vi "Dashboard Main.vi"() -> ()   [LabVIEW 2013]
uses:
  <vilib>/event_ctls.llb/eventvkey.ctl
  <vilib>/Rock Robotics/WPI/Dashboard/WPI_DashboardLogging Global.vi
  <vilib>/Utility/config.llb/Write Key (String).vi
  <vilib>/Utility/config.llb/Write Key (I32).vi
  <vilib>/Utility/config.llb/NI_LVConfig.lvlib
panel:
  out "Image Message":string="Timeout in Camera Communications"
  in  "Rec Mode":enum32{"Stop", "Record", "Playback"}(radio)
  in  "Dashboard Tab":T1(tab)
  out "Limit Switches":T2
  in  "Camera Settings":T3={"Frame Rate"=30, "Compression"=30, "Size"=1} {"Frame Rate" scale=1.0..30.0; "Size" items=["640x480", "320x240", "160x120"]}
  out "MotorSliders R":cluster{"MotorSlide1":dbl, "MotorSlide2":dbl} {"MotorSlide2" scale=-1.0..1.0 scale format="%#_2e"; "MotorSlide1" scale=-1.0..1.0 scale format="%#_2e"}
  out "MotorChart R":cluster{"Numeric":dbl, "Numeric":dbl}(graph)
  out "MotorSliders L":T4 {"MotorSlide4 2" scale=0.0..14.0 scale format="%#_2e"; "MotorSlide2" scale=-1.0..1.0 scale format="%#_2e"; "MotorSlide1" scale=-1.0..1.0 scale format="%#_2e"}
  out "MotorChart L":T5(graph)
  out "JS1 Z":dbl(slide) scale=-1.0..1.0 scale format="%#_2e"
  out "Joystick 1":cluster{"X":dbl, "Y":dbl}[](graph)
  out "JS Buttons 1":T6
  out "JS2 Z":dbl(slide) scale=-1.0..1.0 scale format="%#_2e"
  out "Joystick 2":cluster{"X":dbl, "Y":dbl}[](graph)
  out "JS Buttons 2":T6
  out "Mode":T7(ring)=enum."Auto Disabled"
  out "Camera IP":string
  in  "DB Camera Config":bool
  out "fps":dbl format="%#.1g"
  out "Mbps":dbl format="%#.1g"
  out "Mbps 2":bool
  out "LED 1":bool
  out "Gamepad JS 1":cluster{"X":dbl, "Y":dbl}[](graph)
  out "Gamepad Buttons":T6
  out "Gamepad Triggers":dbl(slide) scale=-1.0..1.0 scale format="%#_2e"
  out "Gamepad JS 2":cluster{"X":dbl, "Y":dbl}[](graph)
  in  "C/J":bool
  in  "T/A":bool
  in  "Slider 1":dbl(slide) scale=0.0..100.0
  in  "Checkbox 2":bool
  in  "Checkbox 1":bool
  in  "Test Slider":dbl(slide) scale=0.0..100.0 scale format="%#_3g"
  in  "On/Off":bool caption="Solenoid"
  in  "Test Name":u16(ring) items=["Select the test to run...", "Example Test", "-------------------------------", "List of tests is built in robot code.", "Replace with your own automated tests."]
  in  "Test Tree":string(tree)
  in  "Motor":cluster{"Value":dbl, "Enable":bool} {"Value" scale=-1.0..1.0 scale format="%#_3g"}
  out "Progress":T8 {"Test Progress" scale=0.0..100.0}
  in  "Rev/Fwd":cluster{"Forward":bool, "Reverse":bool}
  in  "Test Ring":u16(ring) items=["Auto", "Fixed indoor", "Fixed outdoor 1", "Fixed outdoor 2", "Fixed fluorescent 1", "Fixed fluorescent 2", "Hold current"]
  in  "Listbox":i32(listbox)
  out "Tree":string(tree)
  out "Camera Image":T9(plugin-control)
  in  "Enable":bool
  # "Gamepad 1"
  # "Joystick 1"
  # "Joystick 2"
  # "Left"
  # "Front"
  # "Right"
  # "Battery"
  # "Customize by placing controls and indicators here and name to\nmatch Dashboard Variables on robot."
  # "This tab is a great place for autonomous settings and validation.\nCustomize by placing controls and indicators here and name to\nmatch Dashboard Variables on robot."
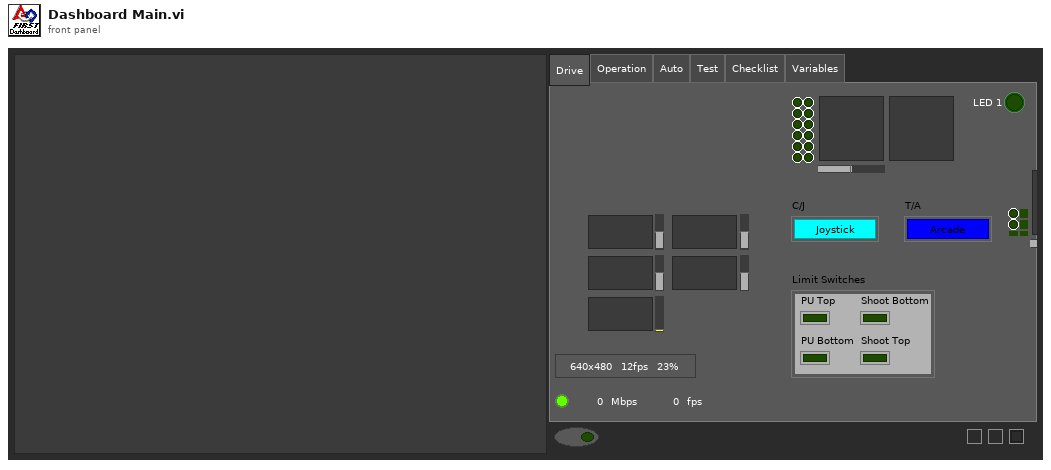
[diagram p1: front panel]
types:
  T1 = enum32{"Drive", "Operation", "Auto", "Test", "Checklist", "Variables"}
  T2 = cluster{"PU Top":bool, "PU Bottom":bool, "Shoot Bottom":bool, "Shoot Top":bool}
  T3 = cluster{"Frame Rate":i32, "Compression":i32, "Size":u16}
  T4 = cluster{"MotorSlide1":dbl, "MotorSlide2":dbl, "MotorSlide4 2":dbl}
  T5 = cluster{"Numeric":dbl, "Numeric":dbl, "Battery":sgl}
  T6 = cluster{bool, bool, bool, bool, bool, bool, bool, bool, bool, bool, bool, bool}
  T7 = enum8{"Tele-Op Disabled", "Tele-Op Enabled", "Auto Disabled", "Auto Enabled", "Test Disabled", "Test Enabled", ""}
  T8 = cluster{"Test Progress":u8, "Test Progress Text":string}
  T9 = typedef "IMAQ Image.ctl" = refnum<image>
  T10 = typedef "Image Type" = u32
  T11 = cluster{"Digital Inputs":bool[], "Digital Outputs":bool[]}
  T12 = cluster{"Competition mode":bool, "Robot Link":bool, "Autonomous":bool, "Enabled":bool, "E-Stop":bool, "Simulated":bool, "TestMode":bool, "Docked Window":bool}
  T13 = cluster{"Boolean Array[0]":bool, "Boolean Array[1]":bool, "Boolean Array[2]":bool, "Boolean Array[3]":bool, "Boolean Array[4]":bool, "Boolean Array[5]":bool, "Boolean Array[6]":bool, "Boolean Array[7]":bool, "Boolean Array[8]":bool, "Boolean Array[9]":bool, "Boolean Array[10]":bool, "Boolean Array[11]":bool}
  T14 = cluster{"Boolean Array[0]":bool, "Boolean Array[1]":bool, "Boolean Array[2]":bool, "Boolean Array[3]":bool}
  T15 = typedef "NI_LVConfig.lvlib/Config Data RefNum.ctl" = refnum<k1>
  T16 = typedef "eventvkey.ctl" = enum16{"ASCII", "Enter", "Return", "Shift", "Ctrl", "Alt", "Cmd", "Opt", "Caps", "NumLock", "Clear", "Break", "Up", "Down", "Left", "Right", "Insert", "Delete", "Home", "End", "PageUp", "PageDown", "Escape", "Help", "Pause", "ScrollLock", "F1", "F2", "F3", "F4", "F5", "F6", "F7", "F8", "F9", "F10", "F11", "F12", "F13", "F14", "F15", "F16", "F17", "F18", "F19", "F20", "F21", "F22", "F23", "F24", "Play", "VolumeUp", "VolumeDown", "Mute", "Two Byte Char"}
  T17 = cluster{"Image Size":bool, "Image Type":bool, "Pixel Value":bool, "ROI Information":bool, "Zoom Factor":bool}
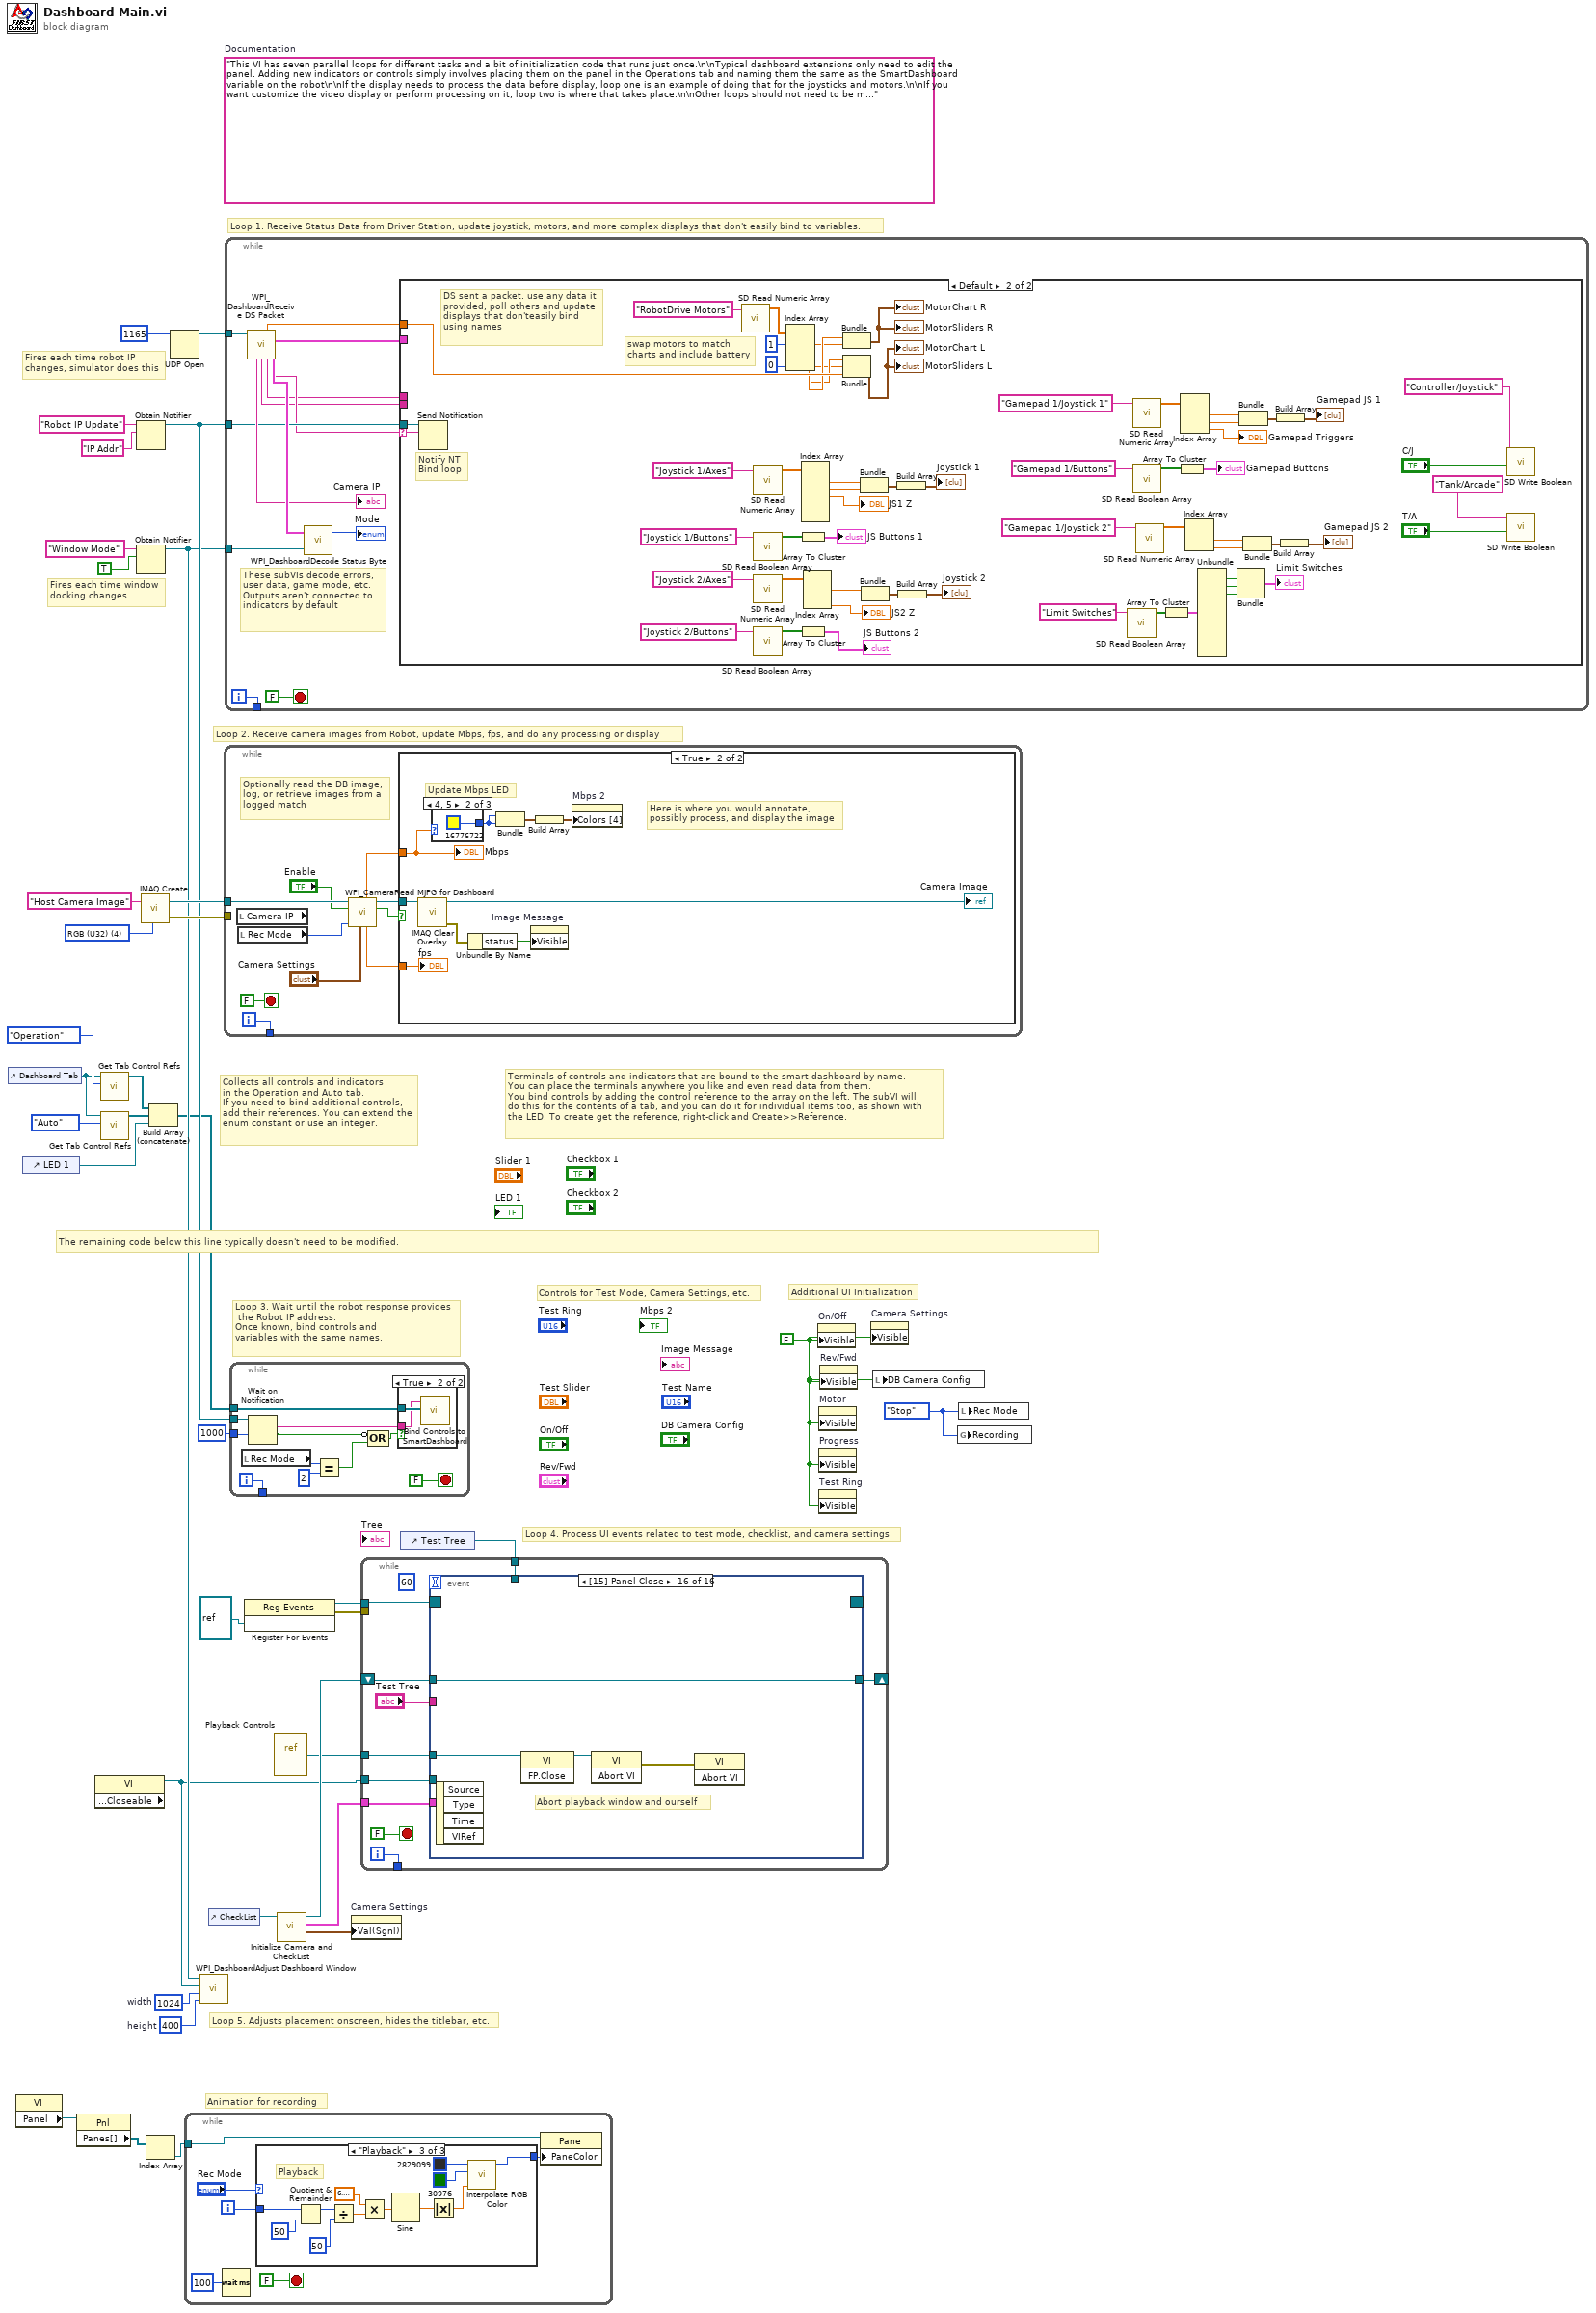
[diagram p0: block diagram]
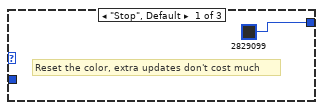
[diagram p2: hidden frame]
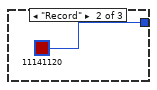
[diagram p3: hidden frame]
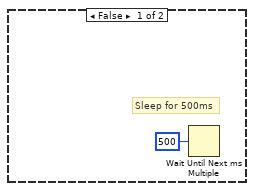
[diagram p5: hidden frame]
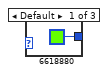
[diagram p6: hidden frame]
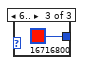
[diagram p7: hidden frame]
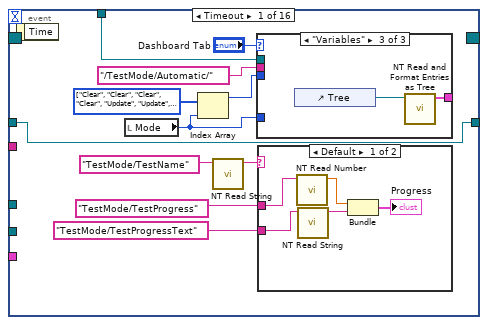
[diagram p8: hidden frame]
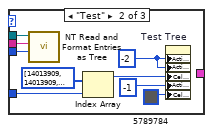
[diagram p10: hidden frame]
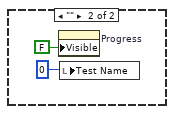
[diagram p11: hidden frame]
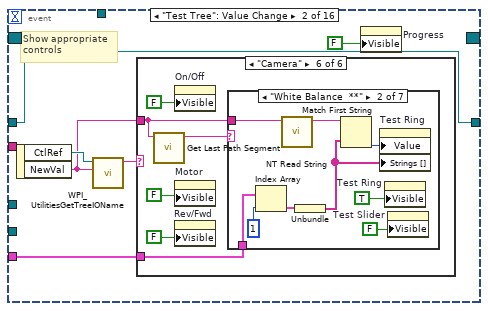
[diagram p12: hidden frame]
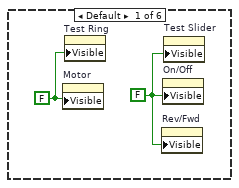
[diagram p13: hidden frame]
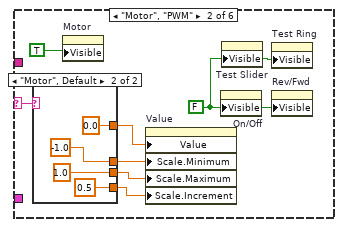
[diagram p14: hidden frame]
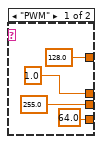
[diagram p15: hidden frame]
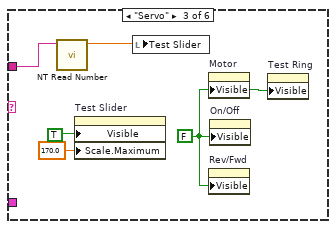
[diagram p16: hidden frame]
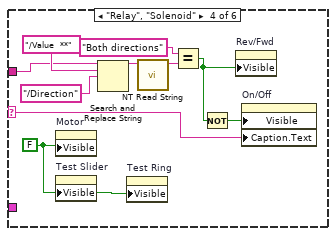
[diagram p17: hidden frame]
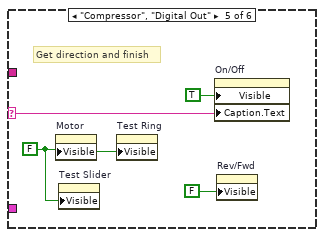
[diagram p18: hidden frame]
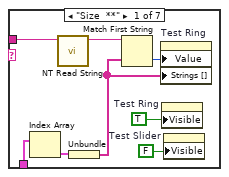
[diagram p19: hidden frame]
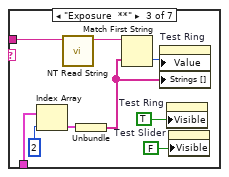
[diagram p20: hidden frame]
diagram:
  w8 = enum32{"Stop", "Record", "Playback"}."Stop" ("Rec Mode")
  w11 = 400  # height
  w12 = 1024  # width
  w25 = FALSE ("Visible")
  (unwired) "This VI has seven parallel loops for different tasks and a bit of initialization code that runs just once.\n\nTypical dashboard extensions only need to edit the panel. Adding new indicators or controls simply involves placing them on the panel in the Operations tab and naming them the same as the SmartDashboard variable on the robot\n\nIf the display needs to process the data before display, loop one is an example of doing that for the joysticks and motors.\n\nIf you want customize the video display or perform processing on it, loop two is where that takes place.\n\nOther loops should not need to be modified. They are pretty standard, and document the task they perform."  # Documentation
  w35 = T10 4 items=["Grayscale (U8)", "Grayscale (I16)", "Grayscale (SGL)", "Complex (CSG)", "RGB (U32)", "HSL (U32)", "RGB (U64)"] ("Image Type")
  # "Controls for Test Mode, Camera Settings, etc."
  # "Additional UI Initialization"
  # "Animation for recording"
  # "Fires each time robot IP\nchanges, simulator does this"
  # "Fires each time window\ndocking changes."
  # "Collects all controls and indicators\nin the Operation and Auto tab.\nIf you need to bind additional controls,\nadd their references. You can extend the\nenum constant or use an integer."
  # "The remaining code below this line typically doesn't need to be modified."
  # "Loop 4. Process UI events related to test mode, checklist, and camera settings"
  # "Terminals of controls and indicators that are bound to the smart dashboard by name.\nYou can place the terminals anywhere you like and even read data from them.\nYou bind controls by adding the control reference to the array on the left. The subVI will\ndo this for the contents of a tab, and you can do it for individual items too, as shown with\nthe LED. To create get the reference, right-click and Create>>Reference."
  # "Loop 3. Wait until the robot response provides\n the Robot IP address.\nOnce known, bind controls and\nvariables with the same names."
  # "Loop 5. Adjusts placement onscreen, hides the titlebar, etc."
  # "Loop 1. Receive Status Data from Driver Station, update joystick, motors, and more complex displays that don't easily bind to variables."
  # "Loop 2. Receive camera images from Robot, update Mbps, fps, and do any processing or display"
  n1 = control-ref of="Dashboard Tab"() -> (w6:refnum<vi>)
  n2 = property class="VI"() -> ("Panel"=w19:refnum<vi>)  [unwired: 2 in, 2 out]
  n3 = control-ref of="LED 1"() -> (w1:refnum<vi>)
  n4 = property class="Pnl"(reference=w19) -> ("Panes[]"=w20:refnum<vi>[])  [unwired: 1 in, 2 out]
  n5 = property class="VI" props=["Front Panel.Closeable"]() -> (reference out=w7:refnum<vi>)  [unwired: 2 in, 2 out]
  n6 = call <vilib>:"Get Tab Control Refs.vi"("Page Index"=T1."Operation" ("Dashboard Tab"), "TabControl in"=w6) -> ("ControlsOnPage"=w4:refnum<vi>[])  [unwired: 9 in]
  n7 = call <vilib>:"Get Tab Control Refs.vi"("Page Index"=T1."Auto" ("Dashboard Tab"), "TabControl in"=w6) -> ("ControlsOnPage"=w5:refnum<vi>[])  [unwired: 9 in]
  n8 = Obtain Notifier(name (unnamed)="Robot IP Update", notification data type="IP Addr" ("name (unnamed)")) -> (notifier out=w29:refnum<notifier>)  [unwired: 2 in, 2 out]
  n9 = Obtain Notifier(name (unnamed)="Window Mode", notification data type=TRUE) -> (notifier out=w10:refnum<notifier>)  [unwired: 2 in, 2 out]
  n10 = call "IMAQ Create"("Image Name"="Host Camera Image", "Image Type"=w35) -> ("New Image"=w33:T9, "error out"=w32:errorcluster)  [unwired: 2 in, 1 out]
  n11 = Index Array(array=w20) -> (element=w18:refnum<vi>)  [unwired: 1 in]
  n12 = Build Array (concatenate)(w4, w5, w1) -> (w3:refnum<vi>[])
  n13 = UDP Open(11:u16 1165 ("port")) -> (port=w36:refnum<k16>)  [unwired: 2 in, 4 out]
  n14 = while {
    tunnel: w18 -> [w39]
    i -> [w42]
    stop <- FALSE stop-if-true
    n15 = Wait (ms)(milliseconds to wait=u32 100) -> ()  [unwired: 1 out]
    n16 = case shown="\"Playback\"" "Rec Mode" {
      tunnel: w42 -> [_ _ w57]
      tunnel: [u32 2829099 ("Base Color") u32 11141120 ("Target Color") w46] -> w38
      frame "Stop", Default {
        # "Reset the color, extra updates don't cost much"
      }
      frame "Record" {
      }
      frame "Playback" {
        # "Playback"
        n17 = Quotient & Remainder(x=w57, y=u32 50 ("milliseconds to wait")) -> (x-y*floor(x/y)=w53:u32)  [unwired: 1 out]
        n18 = Divide(x=w53, y=u32 50 ("milliseconds to wait")) -> (x/y=w50:dbl)
        n19 = Multiply(x=6.283185307179586, y=w50) -> (x*y=w55:dbl)
        n20 = Sine(x=w55) -> (sin(x)=w54:dbl)
        n21 = Absolute Value(x=w54) -> (abs(x)=w47:dbl)
        n22 = call "Interpolate RGB Color.vi"("Proportion"=w47, "Target Color"=u32 30976, "Base Color"=u32 2829099) -> ("Result Color"=w46:u32)  [unwired: 8 in]
      }
    }
    n23 = property class="Pane"(reference=w39, "PaneColor"=w38) -> ()  [unwired: 1 in, 2 out]
  }
  n24 = call <vilib>:"WPI_DashboardAdjust Dashboard Window.vi"("height"=w11, "width"=w12, "reference in"=w7, "Notifier in"=w10) -> ()  [unwired: 8 in]
  n25 = control-ref of="CheckList"() -> (w9:refnum<vi>)
  n26 = while {
    tunnel: w33 -> [w66]
    tunnel: w32 -> [_]
    tunnel: [w67] -> _
    i -> [w67]
    stop <- FALSE stop-if-true
    # "Optionally read the DB image,\nlog, or retrieve images from a\nlogged match"
    n27 = local read "Camera IP"() -> (w59:string)
    n28 = local read "Rec Mode"() -> (w58:enum32{"Stop", "Record", "Playback"})
    n29 = call <vilib>:"WPI_CameraRead MJPG for Dashboard.vi"("Camera Settings"="Camera Settings", "Rec Mode"=w58, "Camera IP"=w59, "Enable"="Enable", "Refnum in"=w66) -> ("Active"=w63:bool, "Refnum out"=w65:T9, "FPS"=w62:dbl, "Bandwidth (Mbps)"=w61:dbl)  [unwired: 3 in]
    n30 = case shown="True" w63 {
      tunnel: w65 -> [_ w73]
      tunnel: w61 -> [_ w72]
      tunnel: w62 -> [_ w70]
      frame False {
        # "Sleep for 500ms"
        n31 = Wait Until Next ms Multiple(millisecond multiple=u32 500) -> ()  [unwired: 1 out]
      }
      frame True {
        # "Here is where you would annotate,\npossibly process, and display the image"
        # "Update Mbps LED"
        n32 = call "IMAQ Clear Overlay"("Image"=w73) -> ("error out"=w77:errorcluster, "Image Out"=→"Camera Image":T9)  [unwired: 2 in, 7 out]
        n33 = case shown="4, 5" w72 {
          tunnel: [u32 6618880 ("Color Box") u32 16776722 ("Color Box") u32 16716800 ("Color Box")] -> w74
          frame Default {
          }
          frame 4, 5 {
          }
          frame 6.. {
          }
        }
        n34 = Unbundle By Name(w77) -> ("status"=w78:bool)
        n35 = Bundle("Color Box"=w74, "Color Box"=w74) -> (w76:cluster{"Color Box":u32, "Color Box":u32})  [unwired: 1 out]
        n36 = property on="Image Message" class="Str"("Visible"=w78) -> ()  [unwired: 2 in, 2 out]
        n37 = Build Array(w76) -> (w75:cluster{"Color Box":u32, "Color Box":u32}[])
        n38 = property on="Mbps 2" class="Bool (strict)"("Colors [4]"=w75) -> ()  [unwired: 2 in, 2 out]
        "Mbps" <- w72
        "fps" <- w70
      }
    }
  }
  n39 = while {
    tunnel: w36 -> [w92]
    tunnel: w29 -> [w87]
    tunnel: w10 -> [w91]
    tunnel: [w88] -> _
    i -> [w88]
    stop <- FALSE stop-if-true
    # "These subVIs decode errors, user data, game mode, etc.\nOutputs aren't connected to indicators by default"
    n40 = call <vilib>:"WPI_DashboardReceive DS Packet.vi"("Recv Socket"=w92) -> ("Battery"=w82:sgl, "Driver Station"=w83:T11, "Robot IP Address"=w86:string, "Status"=w93:T12, "Camera IP Address"=→"Camera IP":string, "Low Priority User Data"=w85:string, "High Priority User Data"=w84:string)  [unwired: 1 in, 7 out]
    n41 = call <vilib>:"WPI_DashboardDecode Status Byte.vi"("Window Mode Notifier"=w91, "Status"=w93) -> ("Mode"=→"Mode":T7)  [unwired: 1 out]
    n42 = case shown="Default" w86 {
      selector: w86 -> [_ w133]
      tunnel: w87 -> [_ w134]
      tunnel: w85 -> [_ _]
      tunnel: w84 -> [_ _]
      tunnel: w83 -> [_ _]
      tunnel: w82 -> [_ w132]
      frame "0.0.0.0" {
        # "DS not sending packets, or no robot exists yet.\nDon't poll the variables"
      }
      frame Default {
        # "Notify NT\nBind loop"
        # "DS sent a packet. use any data it\nprovided, poll others and update\ndisplays that don'teasily bind\nusing names"
        # "swap motors to match\ncharts and include battery"
        n43 = Send Notification(notification=w133, notifier=w134) -> ()  [unwired: 1 in, 2 out]
        n44 = call <vilib>:"SD Read Numeric Array.vi"("Name"="RobotDrive Motors") -> ("Numeric Array"=w131:dbl[])  [unwired: 8 in, 2 out]
        n45 = call <vilib>:"SD Read Numeric Array.vi"("Name"="Joystick 1/Axes") -> ("Numeric Array"=w150:dbl[])  [unwired: 8 in, 2 out]
        n46 = call <vilib>:"SD Read Boolean Array.vi"("Name"="Joystick 1/Buttons") -> ("Boolean Array"=w152:bool[])  [unwired: 8 in, 2 out]
        n47 = call <vilib>:"SD Read Numeric Array.vi"("Name"="Joystick 2/Axes") -> ("Numeric Array"=w144:dbl[])  [unwired: 8 in, 2 out]
        n48 = call <vilib>:"SD Read Boolean Array.vi"("Name"="Joystick 2/Buttons") -> ("Boolean Array"=w143:bool[])  [unwired: 8 in, 2 out]
        n49 = Index Array(array=w131, index #1=1, index #4=0) -> (element #1=w127:dbl, element #2=w126:dbl, element #3=w128:dbl, element #4=w123:dbl)  [unwired: 2 in]
        n50 = Array To Cluster(array=w152) -> (cluster=→"JS Buttons 1":T13)
        n51 = Array To Cluster(array=w143) -> (cluster=→"JS Buttons 2":T13)
        n52 = Index Array(array=w150) -> (element #1=w147:dbl, element #2=w148:dbl, element #3=→"JS1 Z":dbl)  [unwired: 6 in, 3 out]
        n53 = Index Array(array=w144) -> (element #1=w139:dbl, element #2=w138:dbl, element #3=→"JS2 Z":dbl)  [unwired: 3 in]
        n54 = Bundle("Numeric"=w128, "Numeric"=w127) -> (→"MotorChart R" →"MotorSliders R":cluster{"Numeric":dbl, "Numeric":dbl})  [unwired: 1 in]
        n55 = Bundle("Numeric"=w126, "Numeric"=w123, "Battery"=w132) -> (→"MotorChart L" →"MotorSliders L":T5)  [unwired: 1 in]
        n56 = Bundle("Numeric"=w147, "Numeric"=w148) -> (w146:cluster{"Numeric":dbl, "Numeric":dbl})  [unwired: 1 in]
        n57 = Bundle("Numeric"=w139, "Numeric"=w138) -> (w140:cluster{"Numeric":dbl, "Numeric":dbl})  [unwired: 1 in]
        n58 = Build Array(w146) -> (→"Joystick 1":cluster{"Numeric":dbl, "Numeric":dbl}[])
        n59 = Build Array(w140) -> (→"Joystick 2":cluster{"Numeric":dbl, "Numeric":dbl}[])
        n60 = call <vilib>:"SD Read Boolean Array.vi"("Name"="Limit Switches") -> ("Boolean Array"=w105:bool[])  [unwired: 8 in, 2 out]
        n61 = call <vilib>:"SD Read Numeric Array.vi"("Name"="Gamepad 1/Joystick 1") -> ("Numeric Array"=w118:dbl[])  [unwired: 8 in, 2 out]
        n62 = call <vilib>:"SD Read Boolean Array.vi"("Name"="Gamepad 1/Buttons") -> ("Boolean Array"=w120:bool[])  [unwired: 8 in, 2 out]
        n63 = call <vilib>:"SD Read Numeric Array.vi"("Name"="Gamepad 1/Joystick 2") -> ("Numeric Array"=w112:dbl[])  [unwired: 8 in, 2 out]
        n64 = Array To Cluster(array=w105) -> (cluster=w104:T13)
        n65 = Array To Cluster(array=w120) -> (cluster=→"Gamepad Buttons":T13)
        n66 = Index Array(array=w118) -> (element #1=w115:dbl, element #2=w116:dbl, element #3=→"Gamepad Triggers":dbl)  [unwired: 3 in]
        n67 = Index Array(array=w112) -> (element #1=w109:dbl, element #2=w108:dbl)  [unwired: 2 in]
        n68 = Unbundle(w104) -> ("Boolean Array[0]"=w103:bool, "Boolean Array[1]"=w102:bool, "Boolean Array[2]"=w101:bool, "Boolean Array[3]"=w100:bool)  [unwired: 8 out]
        n69 = Bundle("Boolean Array[0]"=w103, "Boolean Array[1]"=w102, "Boolean Array[2]"=w101, "Boolean Array[3]"=w100) -> (→"Limit Switches":T14)  [unwired: 1 in]
        n70 = Bundle("Numeric"=w115, "Numeric"=w116) -> (w114:cluster{"Numeric":dbl, "Numeric":dbl})  [unwired: 1 in]
        n71 = Bundle("Numeric"=w109, "Numeric"=w108) -> (w110:cluster{"Numeric":dbl, "Numeric":dbl})  [unwired: 1 in]
        n72 = Build Array(w114) -> (→"Gamepad JS 1":cluster{"Numeric":dbl, "Numeric":dbl}[])
        n73 = Build Array(w110) -> (→"Gamepad JS 2":cluster{"Numeric":dbl, "Numeric":dbl}[])
        n74 = call <vilib>:"SD Write Boolean.vi"("Boolean"="C/J", "Name"="Controller/Joystick") -> ()  [unwired: 8 in, 2 out]
        n75 = call <vilib>:"SD Write Boolean.vi"("Boolean"="T/A", "Name"="Tank/Arcade") -> ()  [unwired: 8 in, 2 out]
      }
    }
  }
  n76 = while {
    tunnel: w3 -> [w166]
    tunnel: w29 -> [w164]
    tunnel: [w162] -> _
    tunnel: u32 1000 ("milliseconds to wait") -> [w161]
    i -> [w162]
    stop <- FALSE stop-if-true
    n77 = local read "Rec Mode"() -> (w157:enum32{"Stop", "Record", "Playback"})
    n78 = Wait on Notification(notifier=w164, timeout in ms (-1)=w161) -> (notification=w163:string, timed out?=w159:bool)  [unwired: 2 in, 2 out]
    n79 = Equal?(x=w157, y=u16 2 ("Rec Mode")) -> (x = y?=w158:bool)
    n80 = Compound Arithmetic op=OR(invert w159, w158) -> (w160:bool)
    n81 = case shown="True" w160 {
      tunnel: w166 -> [_ w168]
      tunnel: w163 -> [_ w167]
      frame False {
      }
      frame True {
        n82 = call <vilib>:"Bind Controls to SmartDashboard.vi"("Bound Control Refs"=w168, "Server IP Address"=w167) -> ()  [unwired: 10 in]
      }
    }
  }
  n83 = register-events(refnum<vi> refnum) -> (reference out=w16:refnum<event-registration>, error out=w15:errorcluster)  [unwired: 2 in]
  n84 = vi-ref "Playback Controls.vi"() -> (w17:refnum<vi>)
  n85 = call "Initialize Camera and CheckList.vi"("ListBox in"=w9) -> ("Cluster"=w23:cluster{"value":i32, "value":i32, "index":i32}, "Array"=w24:cluster{string[]}[], "File Refnum"=w22:T15)  [unwired: 8 in]
  n86 = property on="Camera Settings" class="Clust (strict)"("Val(Sgnl)"=w23) -> ()  [unwired: 2 in, 2 out]
  n87 = control-ref of="Test Tree"() -> (w21:refnum<vi>)
  n88 = while {
    tunnel: w24 -> [w176]
    shift-right: [w175] -> _
    shift-left: w22 -> [w174]
    tunnel: [w173] -> _
    tunnel: w21 -> [w172]
    tunnel: w17 -> [w171]
    tunnel: w16 -> [w170]
    tunnel: w15 -> [_]
    tunnel: w7 -> [w169]
    i -> [w173]
    stop <- FALSE stop-if-true
    n89 = event shown="[15] Panel Close" {
      selector: w170 -> [_ _ _ _ _ _ _ _ _ _ _ _ _ _ _ _]
      dyn-events: [_ _ _ _ _ _ _ _ _ _ _ _ _ w414 _ _] -> _
      timeout: u32 60 ("milliseconds to wait") -> [_ _ _ _ _ _ _ _ _ _ _ _ _ _ _ _]
      tunnel: w172 -> [w186 _ _ _ _ _ _ _ _ _ _ _ _ _ _ _]
      tunnel: "Test Tree" -> [_ _ _ _ _ _ _ _ w383 w391 w393 w397 w405 _ _ _]
      tunnel: w176 -> [_ w210 _ _ _ _ w347 w377 _ _ _ _ _ _ _ _]
      tunnel: [w180 w209 w308 w313 w321 w333 w346 w370 w382 w389 w392 w396 w404 w416 w430 w431] -> w175
      tunnel: w174 -> [w180 w209 w308 w313 w321 w333 w345 w370 w382 w389 w392 w396 w404 w416 w430 w431]
      tunnel: w171 -> [_ _ _ _ _ _ _ _ _ _ _ _ _ w417 _ w434]
      tunnel: w169 -> [_ _ _ _ _ _ _ _ _ _ _ _ _ w412 _ _]
      event Timeout {
        w185 = enum16{"Update", "Clear"}[] [enum."Clear", enum."Clear", enum."Clear", enum."Clear", enum."Update", enum."Update", enum."Clear"] items=["Update", "Clear"]
        n90 = event-data() -> ()  [unwired: 1 in, 1 out]
        n91 = local read "Mode"() -> (w183:T7)
        n92 = Index Array(array=w185, index=w183) -> (element=w184:enum16{"Update", "Clear"})
        n93 = call <vilib>:"NT Read String.vi"("Name"="TestMode/TestName") -> ("String"=w189:string)  [unwired: 9 in, 1 out]
        n94 = case shown="\"Variables\"" "Dashboard Tab" {
          tunnel: w186 -> [_ w199 _]
          tunnel: "/TestMode/Automatic/" ("Name Pattern") -> [_ w198 _]
          tunnel: w184 -> [_ w197 _]
          tunnel: w183 -> [_ w195 _]
          tunnel: [_ _ w201] -> _
          frame "Operation", Default {
          }
          frame "Test" {
            w194 = -2 ("Active Item:Row Number")
            n95 = call <vilib>:"NT Read and Format Entries as Tree.vi"("Operation"=w197, "Name Pattern"=w198, "Tree Refnum"=w199) -> ()  [unwired: 7 in, 2 out]
            n96 = Index Array(array=u32[] [14013909, 14013909, 14013909, 14013909, 14013909, 16777215, 14013909], index=w195) -> (element=w193:u32)
            n97 = property on="Test Tree" class="Tree (strict)"("Active Item Row Number"=w194, "ActiveColNum"=w194, "CellBG"=w193, "Active Item Row Number"=-1 ("Active Item:Row Number"), "CellBG"=u32 5789784 ("Color Box")) -> ()  [unwired: 2 in, 2 out]
          }
          frame "Variables" {
            n98 = control-ref of="Tree"() -> (w200:refnum<vi>)
            n99 = call <vilib>:"NT Read and Format Entries as Tree.vi"("Tree Refnum"=w200) -> ("Formatted Strings"=w201:cluster{"Name":string, "Value":string}[])  [unwired: 9 in, 1 out]
          }
        }
        n100 = case shown="Default" w189 {
          tunnel: "TestMode/TestProgress" ("Name") -> [w203 _]
          tunnel: "TestMode/TestProgressText" ("Name") -> [w202 _]
          frame Default {
            n101 = call <vilib>:"NT Read Number.vi"("Name"=w203) -> ("Numeric"=w204:dbl)  [unwired: 9 in, 1 out]
            n102 = call <vilib>:"NT Read String.vi"("Name"=w202) -> ("String"=w205:string)  [unwired: 9 in, 1 out]
            n103 = Bundle("Numeric"=w204, "String"=w205) -> (→"Progress":cluster{"Numeric":dbl, "String":string})  [unwired: 1 in]
          }
          frame "" {
            n104 = property on="Progress" class="Clust (strict)"("Visible"=FALSE) -> ()  [unwired: 2 in, 2 out]
            n105 = local write "Test Name"(u16 0) -> ()
          }
        }
      }
      event "Test Tree": Value Change {
        # "Show appropriate\ncontrols"
        n106 = event-data() -> ("CtlRef"=w213:refnum<vi>, "NewVal"=w211:string)  [unwired: 1 in]
        n107 = call <vilib>:"WPI_UtilitiesGetTreeIOName.vi"("NewVal"=w211, "TreeControl in"=w213) -> ("I/O Name"=w214:string)  [unwired: 9 in]
        n108 = case shown="\"Camera\"" w214 {
          selector: w214 -> [_ w221 _ w239 w248 _]
          tunnel: w211 -> [_ _ w236 w238 _ w255]
          tunnel: w210 -> [_ _ _ _ _ w254]
          frame Default {
            w216 = FALSE ("Visible")
            w215 = FALSE ("Visible")
            n109 = property on="Motor" class="Clust (strict)"("Visible"=w215) -> ()  [unwired: 2 in, 2 out]
            n110 = property on="Test Ring" class="Ring (strict)"("Visible"=w215) -> ()  [unwired: 2 in, 2 out]
            n111 = property on="Rev/Fwd" class="Clust (strict)"("Visible"=w216) -> ()  [unwired: 2 in, 2 out]
            n112 = property on="On/Off" class="Bool (strict)"("Visible"=w216) -> ()  [unwired: 2 in, 2 out]
            n113 = property on="Test Slider" class="Slide (strict)"("Visible"=w216) -> ()  [unwired: 2 in, 2 out]
          }
          frame "Motor", "PWM" {
            w222 = FALSE ("Visible")
            n114 = case shown="\"Motor\", Default" w221 {
              tunnel: [1.0 ("Value") -1.0 ("Value")] -> w220
              tunnel: [255.0 ("Value") 1.0 ("Value")] -> w219
              tunnel: [128.0 ("Value") 0.0 ("Value")] -> w218
              tunnel: [64.0 ("Value") 0.5 ("Value")] -> w217
              frame "PWM" {
              }
              frame "Motor", Default {
              }
            }
            n115 = property on="Motor" class="Clust (strict)"("Visible"=TRUE) -> ()  [unwired: 2 in, 2 out]
            n116 = property on="Value" class="Slide (strict)"("Value"=w218, "Scale.Minimum"=w220, "Scale.Maximum"=w219, "Scale.Increment"=w217) -> ()  [unwired: 2 in, 2 out]
            n117 = property on="On/Off" class="Bool (strict)"("Visible"=w222) -> ()  [unwired: 2 in, 2 out]
            n118 = property on="Test Slider" class="Slide (strict)"("Visible"=w222) -> ()  [unwired: 2 in, 2 out]
            n119 = property on="Test Ring" class="Ring (strict)"("Visible"=w222) -> ()  [unwired: 2 in, 2 out]
            n120 = property on="Rev/Fwd" class="Clust (strict)"("Visible"=w222) -> ()  [unwired: 2 in, 2 out]
          }
          frame "Servo" {
            w234 = FALSE ("Visible")
            n121 = call <vilib>:"NT Read Number.vi"("Name"=w236) -> ("Numeric"=w235:dbl)  [unwired: 9 in, 1 out]
            n122 = property on="Test Slider" class="Slide (strict)"("Visible"=TRUE, "Scale.Maximum"=170.0 ("Scale.Range:Maximum")) -> ()  [unwired: 2 in, 2 out]
            n123 = local write "Test Slider"(w235) -> ()
            n124 = property on="Motor" class="Clust (strict)"("Visible"=w234) -> ()  [unwired: 2 in, 2 out]
            n125 = property on="Rev/Fwd" class="Clust (strict)"("Visible"=w234) -> ()  [unwired: 2 in, 2 out]
            n126 = property on="On/Off" class="Bool (strict)"("Visible"=w234) -> ()  [unwired: 2 in, 2 out]
            n127 = property on="Test Ring" class="Ring (strict)"("Visible"=w234) -> ()  [unwired: 2 in, 2 out]
          }
          frame "Relay", "Solenoid" {
            w237 = FALSE ("Visible")
            n128 = property on="Motor" class="Clust (strict)"("Visible"=w237) -> ()  [unwired: 2 in, 2 out]
            n129 = property on="Test Slider" class="Slide (strict)"("Visible"=w237) -> ()  [unwired: 2 in, 2 out]
            n130 = Search and Replace String(input string=w238, search string="/Value  **", replace string="/Direction") -> (result string=w244:string)  [unwired: 5 in, 3 out]
            n131 = property on="Test Ring" class="Ring (strict)"("Visible"=w237) -> ()  [unwired: 2 in, 2 out]
            n132 = call <vilib>:"NT Read String.vi"("Name"=w244) -> ("String"=w242:string)  [unwired: 9 in, 1 out]
            n133 = Equal?(x="Both directions", y=w242) -> (x = y?=w240:bool)
            n134 = Not(x=w240) -> (.not. x?=w241:bool)
            n135 = property on="Rev/Fwd" class="Clust (strict)"("Visible"=w240) -> ()  [unwired: 2 in, 2 out]
            n136 = property on="On/Off" class="Bool (strict)"("Visible"=w241, "Caption.Text"=w239) -> ()  [unwired: 2 in, 2 out]
          }
          frame "Compressor", "Digital Out" {
            w247 = FALSE ("Visible")
            # "Get direction and finish"
            n137 = property on="Motor" class="Clust (strict)"("Visible"=w247) -> ()  [unwired: 2 in, 2 out]
            n138 = property on="Test Slider" class="Slide (strict)"("Visible"=w247) -> ()  [unwired: 2 in, 2 out]
            n139 = property on="Test Ring" class="Ring (strict)"("Visible"=w247) -> ()  [unwired: 2 in, 2 out]
            n140 = property on="On/Off" class="Bool (strict)"("Visible"=TRUE, "Caption.Text"=w248) -> ()  [unwired: 2 in, 2 out]
            n141 = property on="Rev/Fwd" class="Clust (strict)"("Visible"=FALSE) -> ()  [unwired: 2 in, 2 out]
          }
          frame "Camera" {
            n142 = call <vilib>:"Get Last Path Segment.vi"("String in"=w255) -> ("String out"=w256:string)  [unwired: 10 in]
            n143 = property on="On/Off" class="Bool (strict)"("Visible"=FALSE) -> ()  [unwired: 2 in, 2 out]
            n144 = property on="Motor" class="Clust (strict)"("Visible"=FALSE) -> ()  [unwired: 2 in, 2 out]
            n145 = property on="Rev/Fwd" class="Clust (strict)"("Visible"=FALSE) -> ()  [unwired: 2 in, 2 out]
            n146 = case shown="\"White Balance  **\"" w256 {
              tunnel: w255 -> [w262 w271 w280 w289 w298 _ w304]
              tunnel: w254 -> [w260 w268 w277 w286 w295 _ _]
              frame "Size  **" {
                n147 = Index Array(array=w260) -> (element=w259:cluster{string[]})  [unwired: 1 in]
                n148 = call <vilib>:"NT Read String.vi"("Name"=w262) -> ("String"=w261:string)  [unwired: 9 in, 1 out]
                n149 = Unbundle(w259) -> (w257:string[])
                n150 = Match First String(2:w257, 3:w261) -> (0:w258:i32)  [unwired: 1 out]
                n151 = property on="Test Ring" class="Ring (strict)"("Value"=w258, "Strings []"=w257) -> ()  [unwired: 2 in, 2 out]
                n152 = property on="Test Ring" class="Ring (strict)"("Visible"=TRUE) -> ()  [unwired: 2 in, 2 out]
                n153 = property on="Test Slider" class="Slide (strict)"("Visible"=FALSE) -> ()  [unwired: 2 in, 2 out]
              }
              frame "White Balance  **" {
                n154 = Index Array(array=w268, index=1) -> (element=w269:cluster{string[]})
                n155 = call <vilib>:"NT Read String.vi"("Name"=w271) -> ("String"=w270:string)  [unwired: 9 in, 1 out]
                n156 = Unbundle(w269) -> (w266:string[])
                n157 = Match First String(2:w266, 3:w270) -> (0:w265:i32)  [unwired: 1 out]
                n158 = property on="Test Ring" class="Ring (strict)"("Value"=w265, "Strings []"=w266) -> ()  [unwired: 2 in, 2 out]
                n159 = property on="Test Ring" class="Ring (strict)"("Visible"=TRUE) -> ()  [unwired: 2 in, 2 out]
                n160 = property on="Test Slider" class="Slide (strict)"("Visible"=FALSE) -> ()  [unwired: 2 in, 2 out]
              }
              frame "Exposure  **" {
                n161 = Index Array(array=w277, index=2) -> (element=w278:cluster{string[]})
                n162 = call <vilib>:"NT Read String.vi"("Name"=w280) -> ("String"=w279:string)  [unwired: 9 in, 1 out]
                n163 = Unbundle(w278) -> (w274:string[])
                n164 = Match First String(2:w274, 3:w279) -> (0:w275:i32)  [unwired: 1 out]
                n165 = property on="Test Ring" class="Ring (strict)"("Value"=w275, "Strings []"=w274) -> ()  [unwired: 2 in, 2 out]
                n166 = property on="Test Ring" class="Ring (strict)"("Visible"=TRUE) -> ()  [unwired: 2 in, 2 out]
                n167 = property on="Test Slider" class="Slide (strict)"("Visible"=FALSE) -> ()  [unwired: 2 in, 2 out]
              }
              frame "Exposure Priority  **" {
                n168 = Index Array(array=w286, index=3) -> (element=w287:cluster{string[]})
                n169 = call <vilib>:"NT Read String.vi"("Name"=w289) -> ("String"=w288:string)  [unwired: 9 in, 1 out]
                n170 = Unbundle(w287) -> (w283:string[])
                n171 = Match First String(2:w283, 3:w288) -> (0:w284:i32)  [unwired: 1 out]
                n172 = property on="Test Ring" class="Ring (strict)"("Value"=w284, "Strings []"=w283) -> ()  [unwired: 2 in, 2 out]
                n173 = property on="Test Ring" class="Ring (strict)"("Visible"=TRUE) -> ()  [unwired: 2 in, 2 out]
                n174 = property on="Test Slider" class="Slide (strict)"("Visible"=FALSE) -> ()  [unwired: 2 in, 2 out]
              }
              frame "Color Enable  **" {
                n175 = Index Array(array=w295, index=4) -> (element=w296:cluster{string[]})
                n176 = call <vilib>:"NT Read String.vi"("Name"=w298) -> ("String"=w297:string)  [unwired: 9 in, 1 out]
                n177 = Unbundle(w296) -> (w292:string[])
                n178 = Match First String(2:w292, 3:w297) -> (0:w293:i32)  [unwired: 1 out]
                n179 = property on="Test Ring" class="Ring (strict)"("Value"=w293, "Strings []"=w292) -> ()  [unwired: 2 in, 2 out]
                n180 = property on="Test Ring" class="Ring (strict)"("Visible"=TRUE) -> ()  [unwired: 2 in, 2 out]
                n181 = property on="Test Slider" class="Slide (strict)"("Visible"=FALSE) -> ()  [unwired: 2 in, 2 out]
              }
              frame Default {
                n182 = property on="Test Ring" class="Ring (strict)"("Visible"=FALSE) -> ()  [unwired: 2 in, 2 out]
                n183 = property on="Test Slider" class="Slide (strict)"("Visible"=FALSE) -> ()  [unwired: 2 in, 2 out]
              }
              frame "Brightness  **", "Color Level  **", "Compression  **", "FPS  **", "Sharpness  **" {
                n184 = call <vilib>:"NT Read Number.vi"("Name"=w304) -> ("Numeric"=w303:dbl)  [unwired: 9 in, 1 out]
                n185 = local write "Test Slider"(w303) -> ()
                n186 = property on="Test Slider" class="Slide (strict)"("Visible"=TRUE, "Scale.Maximum"=100.0 ("Scale.Range:Maximum")) -> ()  [unwired: 2 in, 2 out]
                n187 = property on="Test Ring" class="Ring (strict)"("Visible"=FALSE) -> ()  [unwired: 2 in, 2 out]
              }
            }
          }
        }
        n188 = property on="Progress" class="Clust (strict)"("Visible"=FALSE) -> ()  [unwired: 2 in, 2 out]
      }
      event "Test Name": Mouse Enter {
        # "Populate the ring with the list of tests"
        n189 = event-data() -> ()  [unwired: 1 in, 1 out]
        n190 = call <vilib>:"NT Read String Array.vi"("Name"="TestMode/TestList") -> ("String Array"=w312:string[])  [unwired: 9 in, 1 out]
        n191 = Build Array (concatenate)("Select the test to run...", w312) -> (w311:string[])
        n192 = property on="Test Name" class="Ring (strict)"("Strings []"=w311) -> ()  [unwired: 2 in, 2 out]
      }
      event "Test Name": Value Change {
        w314 = FALSE ("Visible")
        # "Tell the robot the test name to run"
        n193 = event-data() -> ("NewVal"=w318:u16)  [unwired: 1 in]
        n194 = property on="Test Name" class="Ring (strict)"() -> ("Strings []"=w319:string[])  [unwired: 2 in, 2 out]
        n195 = local write "Progress"(T8 {"Test Progress"=0, "Test Progress Text"=""} ("Progress")) -> ()
        n196 = Index Array(array=w319, index=w318) -> (element=w317:string)
        n197 = call <vilib>:"NT Write String.vi"("String"=w317, "Name"="TestMode/TestName") -> ()  [unwired: 9 in, 1 out]
        n198 = property on="Progress" class="Clust (strict)"("Visible"=TRUE) -> ()  [unwired: 2 in, 2 out]
        n199 = property on="Motor" class="Clust (strict)"("Visible"=w314) -> ()  [unwired: 2 in, 2 out]
        n200 = property on="Test Slider" class="Slide (strict)"("Visible"=w314) -> ()  [unwired: 2 in, 2 out]
        n201 = property on="On/Off" class="Bool (strict)"("Visible"=w314) -> ()  [unwired: 2 in, 2 out]
        n202 = property on="Rev/Fwd" class="Clust (strict)"("Visible"=w314) -> ()  [unwired: 2 in, 2 out]
        n203 = property on="Test Ring" class="Ring (strict)"("Visible"=w314) -> ()  [unwired: 2 in, 2 out]
      }
      event "Listbox": Double Click {
        n204 = event-data() -> ("PlatMods.Shift"=w322:bool, "Row"=w324:i32)  [unwired: 1 in]
        n205 = case shown="True" w322 {
          tunnel: w324 -> [w328 _]
          tunnel: 1 -> [w327 _]
          frame False {
            n206 = property on="Listbox" class="LstBox (strict)"() -> ("Item Symbols"=w326:i32[])  [unwired: 2 in, 2 out]
            n207 = Replace Array Subset(array=w326, new element=w327, index=w328) -> (w325:i32[])
            n208 = property on="Listbox" class="LstBox (strict)"("Item Symbols"=w325) -> ()  [unwired: 2 in, 2 out]
          }
          frame True {
            w329 = 0 ("Top Row")
            n209 = property on="Listbox" class="LstBox (strict)"() -> ("Number of Rows"=w331:u32)  [unwired: 2 in, 2 out]
            n210 = Initialize Array(0, w331) -> (w330:i32[])
            n211 = property on="Listbox" class="LstBox (strict)"("Top Row"=w329, "Value"=w329, "Item Symbols"=w330) -> ()  [unwired: 2 in, 2 out]
          }
        }
      }
      event "Listbox": Key Down {
        n212 = event-data() -> ("VKey"=w335:T16)  [unwired: 1 in]
        n213 = case shown="\"Left\", \"Right\"" w335 {
          selector: w335 -> [w340 _]
          tunnel: eventvkey."Left" ("VKey") -> [w338 _]
          frame "Left", "Right" {
            n214 = Equal?(x=w338, y=w340) -> (x = y?=w339:bool)
            n215 = Select(t=0, s=w339, f=1) -> (s? t:f=w341:i32)
            n216 = property on="Listbox" class="LstBox (strict)"() -> ("Item Symbols"=w344:i32[])  [unwired: 2 in, 2 out]
            n217 = Replace Array Subset(array=w344, new element=w341, index="Listbox") -> (w343:i32[])
            n218 = property on="Listbox" class="LstBox (strict)"("Item Symbols"=w343) -> ()  [unwired: 2 in, 2 out]
          }
          frame Default {
          }
        }
      }
      event "DB Camera Config": Value Change {
        n219 = event-data() -> ("NewVal"=w348:bool)  [unwired: 1 in]
        n220 = case shown="False" w348 {
          tunnel: w347 -> [w357 _]
          tunnel: [w350 w368] -> w346
          tunnel: w345 -> [w349 w368]
          frame False {
            w364 = "Camera"
            w367 = FALSE ("Visible")
            n221 = local read "Camera Settings"() -> (w356:T3)
            n222 = Index Array(array=w357) -> (element=w360:cluster{string[]})  [unwired: 1 in]
            n223 = Unbundle(w356) -> ("Frame Rate"=w355:i32, "Compression"=w354:i32, "Size"=w358:u16)
            n224 = Unbundle(w360) -> (w359:string[])
            n225 = Index Array(array=w359, index=w358) -> (element=w353:string)
            n226 = call-poly <vilib>:"Write Key.vi"("section"=w364, "value"=w353, "key"="Size", "refnum"=w349) -> ("refnum out"=w366:T15)  [unwired: 2 in, 5 out]
            n227 = call-poly <vilib>:"Write Key.vi"("section"=w364, "value"=w355, "key"="FrameRate", "refnum"=w366) -> ("refnum out"=w365:T15)  [unwired: 1 in, 6 out]
            n228 = property on="Camera Settings" class="Clust (strict)"("Visible"=w367) -> ()  [unwired: 2 in, 2 out]
            n229 = local write "DB Camera Config"(w367) -> ()
            n230 = call-poly <vilib>:"Write Key.vi"("section"=w364, "value"=w354, "key"="Compression", "refnum"=w365) -> ("refnum out"=w351:T15)  [unwired: 1 in, 6 out]
            n231 = call <vilib>:"Close Config Data.vi"("refnum"=w351) -> ("file path"=w352:path)  [unwired: 2 in, 8 out]
            n232 = call <vilib>:"Open Config Data.vi"("configuration file path"=w352) -> ("refnum"=w350:T15)  [unwired: 8 in, 2 out]
          }
          frame True {
            n233 = property on="Camera Settings" class="Clust (strict)"("Visible"=TRUE) -> ()  [unwired: 2 in, 2 out]
          }
        }
      }
      event "Camera Settings": Value Change {
        n234 = event-data() -> ("NewVal"=w381:T3)  [unwired: 1 in]
        n235 = Index Array(array=w377) -> (element=w376:cluster{string[]})  [unwired: 1 in]
        n236 = Unbundle(w381) -> ("Frame Rate"=w372:i32, "Compression"=w371:i32, "Size"=w374:u16)
        n237 = Unbundle(w376) -> (w375:string[])
        n238 = Index Array(array=w375, index=w374) -> (element=w373:string)
        n239 = Format Into String(format string="%s   %dfps   %d%%", w373, w372, w371) -> (resulting string=w378:string)  [unwired: 2 in, 1 out]
        n240 = Build Array(w378) -> (w379:string[])
        n241 = property on="DB Camera Config" class="Bool (strict)"("Strings [4]"=w379) -> ()  [unwired: 2 in, 2 out]
      }
      event "Motor.Enable": Value Change {
        n242 = event-data() -> ("NewVal"=w387:bool)  [unwired: 1 in]
        n243 = Unbundle("Motor") -> ("Value"=w386:dbl)  [unwired: 1 out]
        n244 = Select(t=w386, s=w387, f=0.0) -> (s? t:f=w384:dbl)
        n245 = call <vilib>:"NT Write Number.vi"("Numeric"=w384, "Name"=w383) -> ()  [unwired: 9 in, 1 out]
      }
      event "Test Slider": Value Change {
        n246 = event-data() -> ("NewVal"=w390:dbl)  [unwired: 1 in]
        n247 = call <vilib>:"NT Write Number.vi"("Numeric"=w390, "Name"=w391) -> ()  [unwired: 9 in, 1 out]
      }
      event "On/Off": Value Change {
        n248 = event-data() -> ("NewVal"=w395:bool)  [unwired: 1 in]
        n249 = Boolean To (0,1)(Boolean=w395) -> (0, 1=w394:i16)
        n250 = call <vilib>:"NT Write Number.vi"("Numeric"=w394, "Name"=w393) -> ()  [unwired: 9 in, 1 out]
      }
      event "Rev/Fwd": Value Change {
        n251 = event-data() -> ("NewVal.Forward"=w403:bool, "NewVal.Reverse"=w402:bool)  [unwired: 1 in]
        n252 = Boolean To (0,1)(Boolean=w403) -> (0, 1=w399:i16)
        n253 = Boolean To (0,1)(Boolean=w402) -> (0, 1=w401:i16)
        n254 = Negate(x=w401) -> (-x=w400:i16)
        n255 = Add(x=w399, y=w400) -> (x+y=w398:i16)
        n256 = call <vilib>:"NT Write Number.vi"("Numeric"=w398, "Name"=w397) -> ()  [unwired: 9 in, 1 out]
      }
      event "Test Ring": Value Change {
        n257 = event-data() -> ("NewVal"=w407:u16)  [unwired: 1 in]
        n258 = property on="Test Ring" class="Ring (strict)"() -> ("Strings []"=w408:string[])  [unwired: 2 in, 2 out]
        n259 = Index Array(array=w408, index=w407) -> (element=w406:string)
        n260 = call <vilib>:"NT Write String.vi"("String"=w406, "Name"=w405) -> ()  [unwired: 9 in, 1 out]
      }
      event "Rec Mode": Value Change {
        # "Update globals for recording mode and path to read log from.\nClear when logging and let NetworkTables set path for vision to\nuse."
        n261 = event-data() -> ("NewVal"=w418:enum32{"Stop", "Record", "Playback"})  [unwired: 1 in]
        n262 = global write "WPI_DashboardLogging Global.vi" "Logging Filename"(path "") -> ()
        n263 = case shown="\"Stop\", \"Record\"" w418 {
          tunnel: w417 -> [_ w420 w428]
          tunnel: [_ _ w427] -> w414
          tunnel: [_ _ w426] -> _
          tunnel: w412 -> [_ _ w424]
          tunnel: cluster{i32, i32} {-250, 170} -> [_ _ w423]
          tunnel: [_ _ T17 {"Image Size"=TRUE, "Image Type"=TRUE, "Pixel Value"=TRUE, "ROI Information"=TRUE, "Zoom Factor"=FALSE} ("Image Information Shown:All Elements")] -> w410
          tunnel: [_ _ TRUE ("Zoom Factor")] -> w409
          frame Default {
          }
          frame "Stop", "Record" {
            # "Place Window too"
            n264 = invoke class="VI" method="FP.Close"(reference=w420) -> (reference out=w419:refnum<vi>)  [unwired: 2 in, 2 out]
            n265 = invoke class="VI" method="Abort VI"(reference=w419) -> ()  [unwired: 2 in, 3 out]
          }
          frame "Playback" {
            n266 = call "Open Playback Panel.vi"("Offset"=w423, "DB VI Ref"=w424, "Playback in"=w428) -> ("Playback out"=w425:refnum<vi>)  [unwired: 8 in]
            n267 = register-events(w425) -> (reference out=w427:refnum<event-registration>, error out=w426:errorcluster)  [unwired: 2 in]
          }
        }
        n268 = global write "WPI_DashboardLogging Global.vi" "Recording"(w418) -> ()
        n269 = property on="Camera Image" class="ImageControl"("Image Information Shown"=w410, "Image Information Visible"=w409) -> ()  [unwired: 2 in, 2 out]
        n270 = call <vilib>:"WPI_DashboardNT Log FieldName Cache.vi"("Operation"=enum16{"Lookup/Add", "Index", "Clear"}."Clear") -> ()  [unwired: 8 in, 3 out]
      }
      event Panel Close {
        w429 = enum32{"Stop", "Record", "Playback"}."Stop" ("Rec Mode")
        n271 = event-data() -> ()  [unwired: 1 in, 4 out]
        n272 = local write "Rec Mode"(w429) -> ()
        n273 = global write "WPI_DashboardLogging Global.vi" "Recording"(w429) -> ()
      }
      event Panel Close {
        # "Abort playback window and ourself"
        n274 = event-data() -> ()  [unwired: 1 in, 4 out]
        n275 = invoke class="VI" method="FP.Close"(reference=w434) -> (reference out=w433:refnum<vi>)  [unwired: 2 in, 2 out]
        n276 = invoke class="VI" method="Abort VI"(reference=w433) -> (error out=w432:errorcluster)  [unwired: 2 in, 2 out]
        n277 = invoke class="VI" method="Abort VI"(error in=w432) -> ()  [unwired: 2 in, 3 out]
      }
    }
  }
  n278 = property on="On/Off" class="Bool (strict)"("Visible"=w25) -> ()  [unwired: 2 in, 2 out]
  n279 = property on="Motor" class="Clust (strict)"("Visible"=w25) -> ()  [unwired: 2 in, 2 out]
  n280 = property on="Progress" class="Clust (strict)"("Visible"=w25) -> ()  [unwired: 2 in, 2 out]
  n281 = property on="Test Ring" class="Ring (strict)"("Visible"=w25) -> ()  [unwired: 2 in, 2 out]
  n282 = property on="Rev/Fwd" class="Clust (strict)"("Visible"=w25) -> ()  [unwired: 2 in, 2 out]
  n283 = property on="Camera Settings" class="Clust (strict)"("Visible"=w25) -> ()  [unwired: 2 in, 2 out]
  n284 = local write "DB Camera Config"(w25) -> ()
  n285 = global write "WPI_DashboardLogging Global.vi" "Recording"(w8) -> ()
  n286 = local write "Rec Mode"(w8) -> ()
